vi "Stop Core.vi"(10 "final error code":i32, 11 "Storage Line in":refnum<class "Storage Line.lvclass">) -> (3 "Storage Line out":refnum<class "Storage Line.lvclass">)   [LabVIEW 2015, in "cRIO-Carbondioxide.lvlib" / "CO2-Actor.lvlib" / "Storage Line.lvclass"]
doc: "(<B>Filename</B>: Actor Framework.lvlib:Actor.lvclass:Stop Core.vi)\n\nDefines what the actor does before it stops. Use the <B>final error code</B> input to determine whether the actor shut down in response to an error.\n\nBy default, this method does nothing. A descendant class may override it to define behavior, such as shutting down any processes the actor initiated in its override of the Actor Core method."
uses:
  Storage Line.lvclass
  Storage Line.lvclass/Storage Line.ctl
  <vilib>/ActorFramework/Message Enqueuer/Message Enqueuer.lvclass/Message Enqueuer.ctl
  <vilib>/ActorFramework/Message Enqueuer/Enqueue.vi
  <vilib>/ActorFramework/Message Priority Queue/Priority Enqueue.vi
  <vilib>/ActorFramework/Stop Msg/Stop Msg.lvclass
  CO2 Actor/CO2 Actor.lvclass
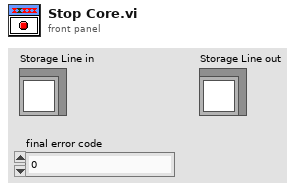
[diagram p1: front panel]
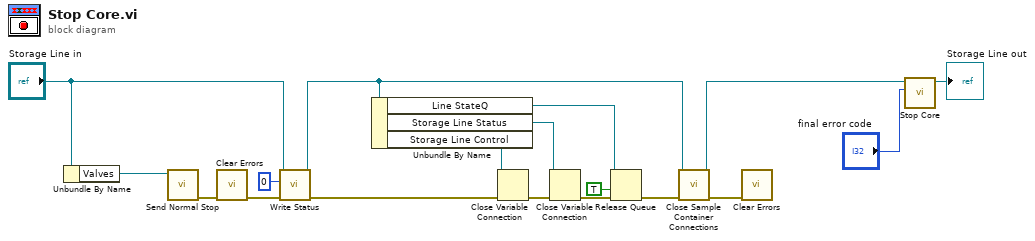
[diagram p0: block diagram]
diagram:
  n1 = Unbundle By Name("Storage Line in") -> ("Valves"=w15:refnum<class "Message Enqueuer.lvclass">)
  n2 = call <vilib>:"Send Normal Stop.vi"("Message Enqueuer"=w15) -> ("error out"=w16:errorcluster)  [unwired: 10 in]
  n3 = call <vilib>:"Clear Errors.vi"("error in (no error)"=w16) -> ("error out"=w11:errorcluster)  [unwired: 5 in, 1 out]
  n4 = call "Write Status.vi"("error in (no error)"=w11, "Status Bitfield"=u16 0 ("Status"), "Storage Line in"="Storage Line in") -> ("error out"=w10:errorcluster, "Storage Line out"=w7:refnum<class "Storage Line.lvclass">)  [unwired: 6 in, 1 out]
  n5 = Unbundle By Name(w7) -> ("Line StateQ"=w3:refnum<queue>, "Storage Line Status"=w12:refnum<k21>, "Storage Line Control"=w14:refnum<k21>)
  n6 = Close Variable Connection(8:w10, 11:w14) -> (0:w13:errorcluster)
  n7 = Close Variable Connection(8:w13, 11:w12) -> (0:w4:errorcluster)
  n8 = Release Queue(queue=w3, force destroy? (F)=TRUE, error in (no error)=w4) -> (error out=w2:errorcluster)  [unwired: 2 out]
  n9 = call "Close Sample Container Connections.vi"("error in (no error)"=w2, "Storage Line in"=w7) -> ("error out"=w5:errorcluster, "Storage Line out"=w6:refnum<class "Storage Line.lvclass">)  [unwired: 8 in]
  n10 = call <vilib>:"Clear Errors.vi"("error in (no error)"=w5) -> ()  [unwired: 5 in, 2 out]
  n11 = call-parent "Stop Core.vi"("final error code"="final error code", "CO2 Actor in"=w6) -> ("CO2 Actor out"=→"Storage Line out":refnum<class "Storage Line.lvclass">)  [unwired: 9 in]
